vi "maincapactor11.vi"() -> ()   [LabVIEW 2020]
panel:
  out "dup directory path":path
  in  "GPIB address magnet":string="1"
  in  "GPIB address Temp Controler":string="12"
  in  "GPIB address CapBridge":string="6"
  in  "Wait (second)":u32
  in  "No of Temp Steps":i16
  in  "folder name to save files":string
  out "outputtemp":dbl[](array[numeric]) format="%.2f"
  out "outputdc":dbl[](array[numeric]) format="%.2f"
  out "outputcapacitor":dbl[](array[numeric]) format="%.2f"
  out "field":dbl[](array[numeric]) format="%.2f"
  out "Current Temp":dbl format="%.3f"
  in  "Increasing \nTemp step":bool=TRUE
  in  "Temperature\nInterval":dbl format="%.3f"
  in  "Initial Temp C":dbl format="%.3f"
  # "Help:\n1. write the folder name to save the files.The file name will \nbe the temperature in the given folder.\n2.Write the GPIB address of all the instruments before running\nthe program.\n3. Give the initial temperature and the temperature interval \nand the total number of steps.\n4.Check whether you want to increase the temperature or\ndecrease.\n5.Write the time to be waited to let the tempetature controller\nequilibrate.\n6.Once the speps 1 through 5 is done run the experiment."
  # "Decreasing\nTemp Step"
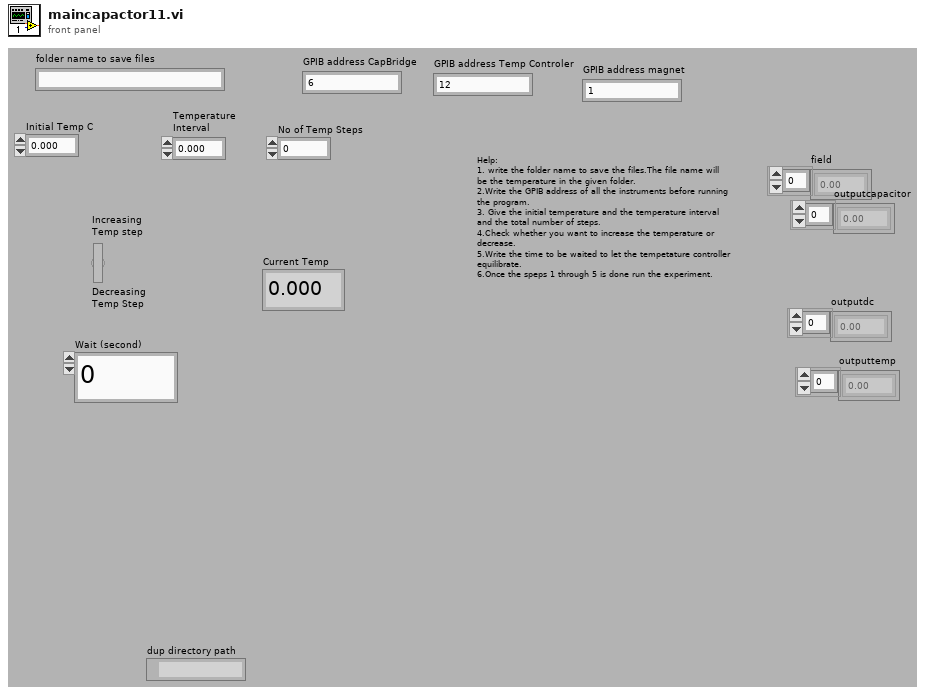
[diagram p1: front panel]
types:
  T1 = enum16{"--Quit--", "Read-Status", "Read-Cell", "Read-Field[T]", "Read-Setpoint[T]"}
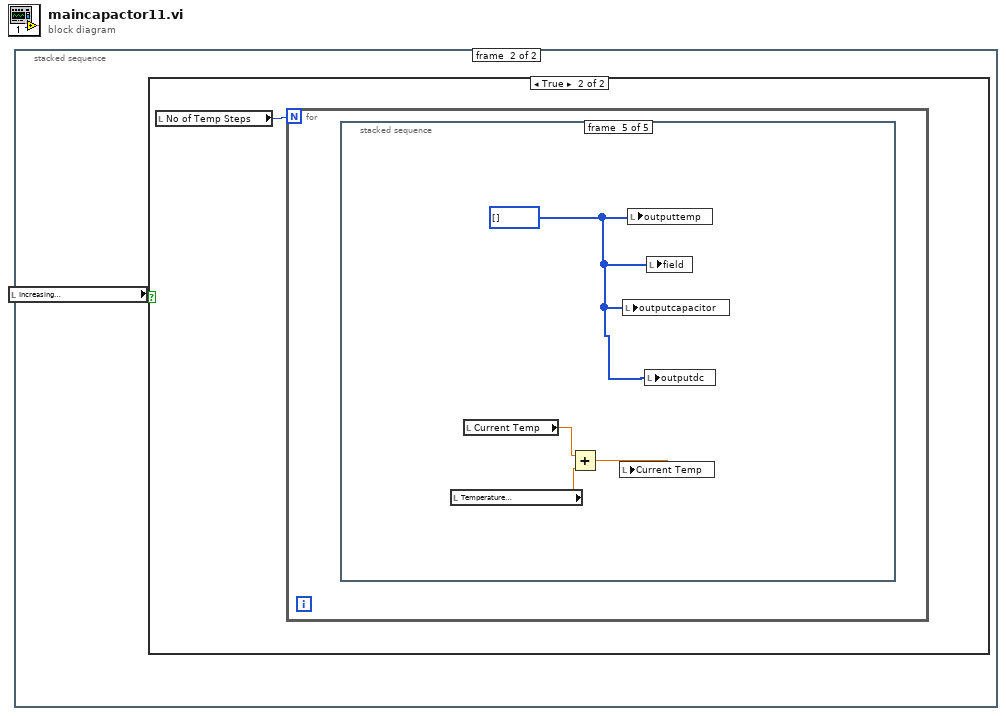
[diagram p0: block diagram]
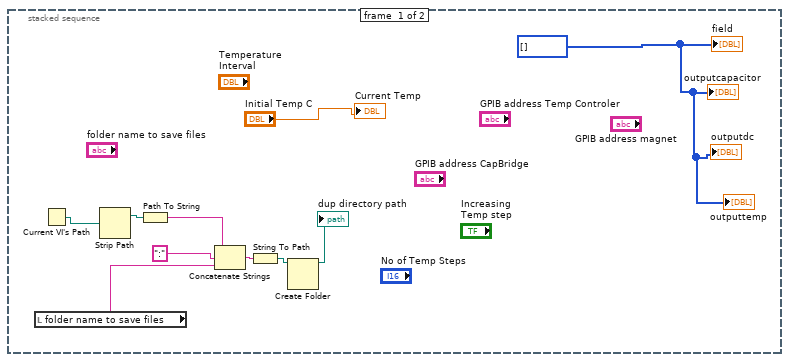
[diagram p2: hidden frame]
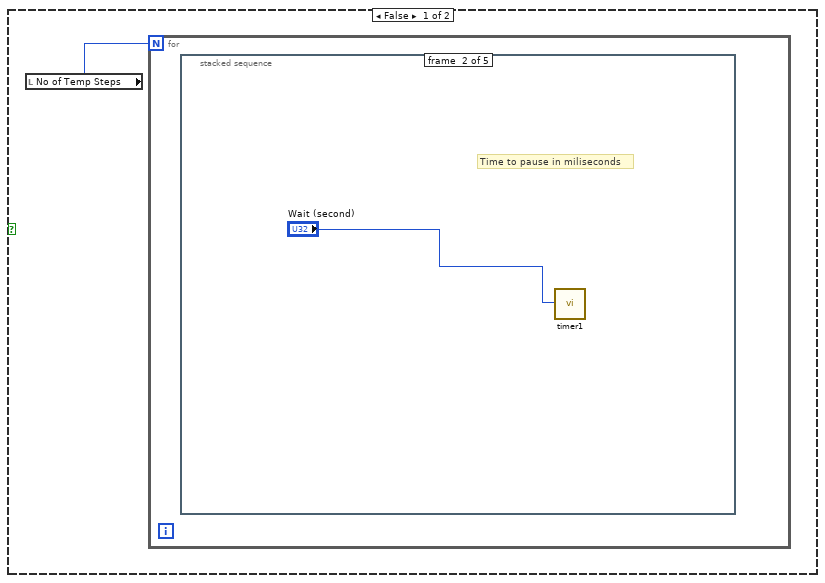
[diagram p3: hidden frame]
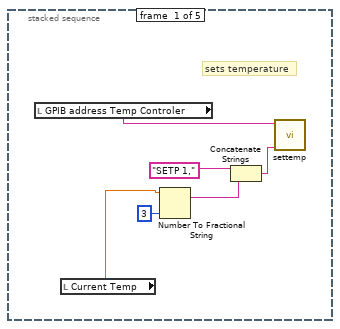
[diagram p4: hidden frame]
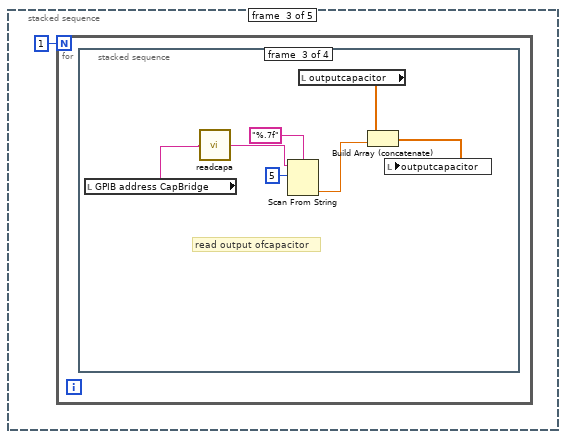
[diagram p5: hidden frame]
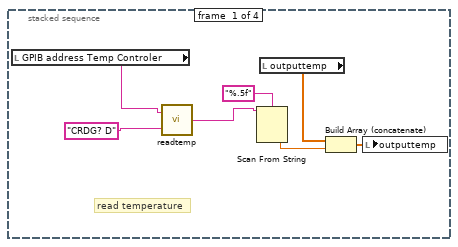
[diagram p6: hidden frame]
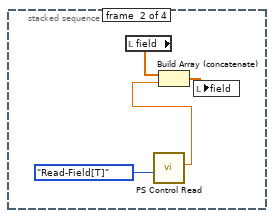
[diagram p7: hidden frame]
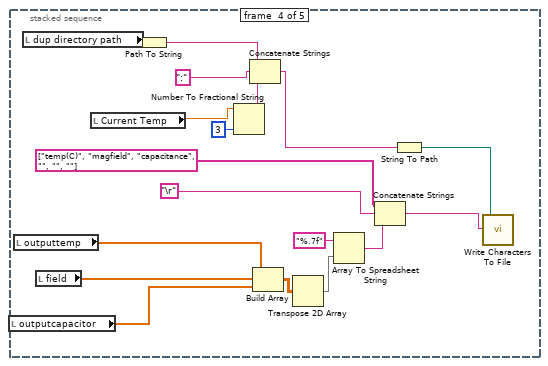
[diagram p9: hidden frame]
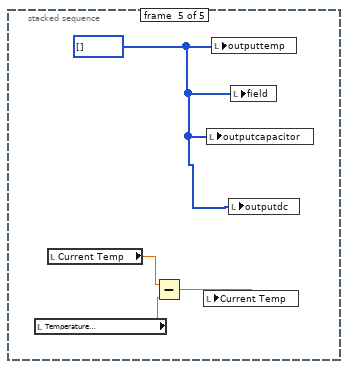
[diagram p10: hidden frame]
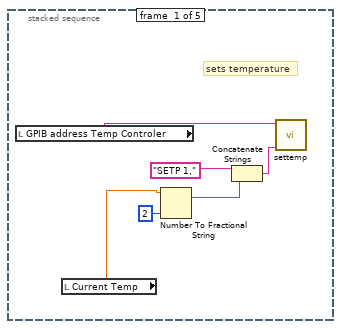
[diagram p11: hidden frame]
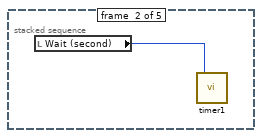
[diagram p12: hidden frame]
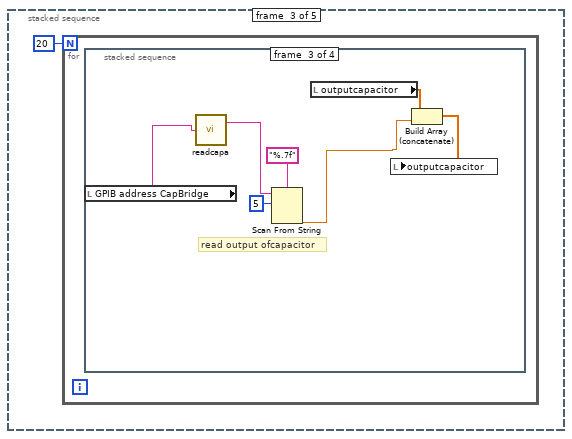
[diagram p13: hidden frame]
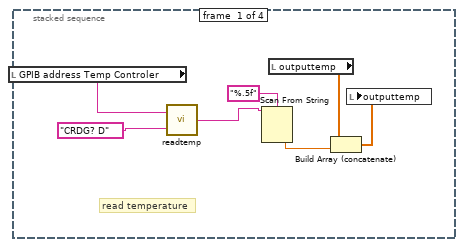
[diagram p14: hidden frame]
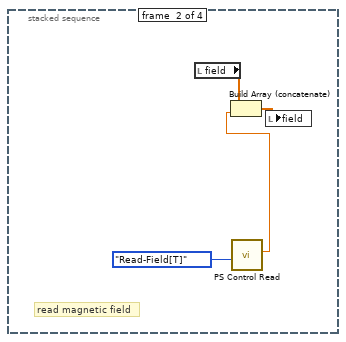
[diagram p15: hidden frame]
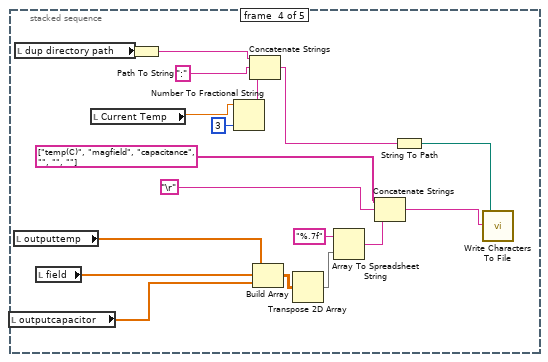
[diagram p17: hidden frame]
diagram:
  n1 = stacked-sequence {
    frame #0 {
      w9 = i32[] [] ("field")
      n2 = local read "folder name to save files"() -> (w4:string)
      n3 = Current VI's Path() -> (path=w8:path)
      n4 = Strip Path(path=w8) -> (stripped path=w7:path)  [unwired: 1 out]
      n5 = Path To String(path=w7) -> (string=w6:string)
      n6 = Concatenate Strings(w6, ":", w4) -> (w3:string)
      n7 = String To Path(string=w3) -> (path=w2:path)
      n8 = Create Folder(path (use dialog)=w2) -> (created path=→"dup directory path":path)  [unwired: 2 in, 2 out]
      "Current Temp" <- "Initial Temp C"
      "field" <- w9
      "outputcapacitor" <- w9
      "outputdc" <- w9
      "outputtemp" <- w9
    }
    frame #1 {
      n9 = local read "Increasing \nTemp step"() -> (w11:bool)
      n10 = case shown="True" w11 {
        frame False {
          n11 = local read "No of Temp Steps"() -> (w12:i16)
          n12 = for {
            N: w12 -> [_]
            n13 = stacked-sequence {
              frame #0 {
                # "sets temperature"
                n14 = local read "GPIB address Temp Controler"() -> (w13:string)
                n15 = local read "Current Temp"() -> (w15:dbl)
                n16 = Number To Fractional String(number=w15, precision (6)=i16 3) -> (F-format string=w18:string)  [unwired: 2 in]
                n17 = Concatenate Strings("SETP 1,", w18) -> (w16:string)
                n18 = call "settemp.vi"("Characters to Write"=w16, "GPIB\nAddress"=w13) -> ()  [unwired: 5 in, 1 out]
              }
              frame #1 {
                # "Time to pause in miliseconds"
                n19 = call "timer1.vi"("Numeric 2"="Wait (second)") -> ()  [unwired: 1 in]
              }
              frame #2 {
                n20 = for {
                  N: 1 -> [_]
                  n21 = stacked-sequence {
                    frame #0 {
                      # "read temperature"
                      n22 = local read "GPIB address Temp Controler"() -> (w23:string)
                      n23 = call "readtemp.vi"("Characters to Write"="CRDG? D", "GPIB\nAddress"=w23) -> ("Characters Read"=w24:string)
                      n24 = Scan From String(format string="%.5f", input string=w24) -> (output 1=w21:dbl)  [unwired: 3 in, 3 out]
                      n25 = local read "outputtemp"() -> (w22:dbl[])
                      n26 = Build Array (concatenate)(w22, w21) -> (w27:dbl[])
                      n27 = local write "outputtemp"(w27) -> ()
                    }
                    frame #1 {
                      n28 = local read "field"() -> (w30:dbl[])
                      n29 = call "PS Control Read.vi"("Read State"=T1."Read-Field[T]") -> ("Current Field"=w28:dbl)  [unwired: 3 in, 4 out]
                      n30 = Build Array (concatenate)(w30, w28) -> (w31:dbl[])
                      n31 = local write "field"(w31) -> ()
                    }
                    frame #2 {
                      # "read output ofcapacitor"
                      n32 = local read "GPIB address CapBridge"() -> (w37:string)
                      n33 = call "readcapa.vi"("GPIB\nAddress"=w37) -> ("Characters Read"=w33:string)
                      n34 = Scan From String(format string="%.7f", input string=w33, initial scan location=u32 5) -> (output 1=w32:dbl)  [unwired: 2 in, 3 out]
                      n35 = local read "outputcapacitor"() -> (w36:dbl[])
                      n36 = Build Array (concatenate)(w36, w32) -> (w38:dbl[])
                      n37 = local write "outputcapacitor"(w38) -> ()
                    }
                    frame #3 {
                      # "pause if needed"
                    }
                  }
                }
              }
              frame #3 {
                n38 = local read "outputcapacitor"() -> (w41:dbl[])
                n39 = local read "outputtemp"() -> (w51:dbl[])
                n40 = local read "dup directory path"() -> (w40:path)
                n41 = local read "field"() -> (w50:dbl[])
                n42 = local read "Current Temp"() -> (w53:dbl)
                n43 = Path To String(path=w40) -> (string=w39:string)
                n44 = Number To Fractional String(number=w53, precision (6)=i16 3) -> (F-format string=w52:string)  [unwired: 2 in]
                n45 = Concatenate Strings(w39, ":", w52) -> (w55:string)
                n46 = Build Array(w51, w50, w41) -> (w49:dbl[][])
                n47 = Transpose 2D Array(2D array=w49) -> (transposed array=w47:dbl[][])
                n48 = Array To Spreadsheet String(array=w47, 3:"%.7f" ("format string")) -> (spreadsheet string=w44:string)  [unwired: 1 in]
                n49 = Concatenate Strings(string[] ["temp(C)", "magfield", "capacitance", "", "", ""], "\r", w44) -> (w43:string)
                n50 = String To Path(string=w55) -> (path=w54:path)
                n51 = call <vilib>:"Write Characters To File.vi"("character string"=w43, "file path (dialog if empty)"=w54) -> ()  [unwired: 3 in, 1 out]
              }
              frame #4 {
                w60 = i32[] []
                n52 = local read "Temperature\nInterval"() -> (w58:dbl)
                n53 = local read "Current Temp"() -> (w59:dbl)
                n54 = Subtract(x=w59, y=w58) -> (x-y=w57:dbl)
                n55 = local write "Current Temp"(w57) -> ()
                n56 = local write "outputcapacitor"(w60) -> ()
                n57 = local write "outputtemp"(w60) -> ()
                n58 = local write "outputdc"(w60) -> ()
                n59 = local write "field"(w60) -> ()
              }
            }
          }
        }
        frame True {
          n60 = local read "No of Temp Steps"() -> (w61:i16)
          n61 = for {
            N: w61 -> [_]
            n62 = stacked-sequence {
              frame #0 {
                # "sets temperature"
                n63 = local read "GPIB address Temp Controler"() -> (w62:string)
                n64 = local read "Current Temp"() -> (w64:dbl)
                n65 = Number To Fractional String(number=w64, precision (6)=i16 2) -> (F-format string=w67:string)  [unwired: 2 in]
                n66 = Concatenate Strings("SETP 1,", w67) -> (w65:string)
                n67 = call "settemp.vi"("Characters to Write"=w65, "GPIB\nAddress"=w62) -> ()  [unwired: 5 in, 1 out]
              }
              frame #1 {
                n68 = local read "Wait (second)"() -> (w68:u32)
                n69 = call "timer1.vi"("Numeric 2"=w68) -> ()  [unwired: 1 in]
              }
              frame #2 {
                n70 = for {
                  N: 20 -> [_]
                  n71 = stacked-sequence {
                    frame #0 {
                      # "read temperature"
                      n72 = local read "GPIB address Temp Controler"() -> (w72:string)
                      n73 = call "readtemp.vi"("Characters to Write"="CRDG? D", "GPIB\nAddress"=w72) -> ("Characters Read"=w73:string)
                      n74 = Scan From String(format string="%.5f", input string=w73) -> (output 1=w70:dbl)  [unwired: 3 in, 3 out]
                      n75 = local read "outputtemp"() -> (w71:dbl[])
                      n76 = Build Array (concatenate)(w71, w70) -> (w76:dbl[])
                      n77 = local write "outputtemp"(w76) -> ()
                    }
                    frame #1 {
                      # "read magnetic field"
                      n78 = local read "field"() -> (w79:dbl[])
                      n79 = call "PS Control Read.vi"("Read State"=T1."Read-Field[T]") -> ("Current Field"=w77:dbl)  [unwired: 3 in, 4 out]
                      n80 = Build Array (concatenate)(w79, w77) -> (w80:dbl[])
                      n81 = local write "field"(w80) -> ()
                    }
                    frame #2 {
                      # "read output ofcapacitor"
                      n82 = local read "GPIB address CapBridge"() -> (w86:string)
                      n83 = call "readcapa.vi"("GPIB\nAddress"=w86) -> ("Characters Read"=w82:string)
                      n84 = Scan From String(format string="%.7f", input string=w82, initial scan location=u32 5) -> (output 1=w81:dbl)  [unwired: 2 in, 3 out]
                      n85 = local read "outputcapacitor"() -> (w85:dbl[])
                      n86 = Build Array (concatenate)(w85, w81) -> (w87:dbl[])
                      n87 = local write "outputcapacitor"(w87) -> ()
                    }
                    frame #3 {
                      # "pause if needed to take readings"
                    }
                  }
                }
              }
              frame #3 {
                n88 = local read "outputcapacitor"() -> (w90:dbl[])
                n89 = local read "outputtemp"() -> (w100:dbl[])
                n90 = local read "dup directory path"() -> (w89:path)
                n91 = local read "field"() -> (w99:dbl[])
                n92 = local read "Current Temp"() -> (w102:dbl)
                n93 = Path To String(path=w89) -> (string=w88:string)
                n94 = Number To Fractional String(number=w102, precision (6)=i16 3) -> (F-format string=w101:string)  [unwired: 2 in]
                n95 = Concatenate Strings(w88, ":", w101) -> (w104:string)
                n96 = Build Array(w100, w99, w90) -> (w98:dbl[][])
                n97 = Transpose 2D Array(2D array=w98) -> (transposed array=w96:dbl[][])
                n98 = Array To Spreadsheet String(array=w96, 3:"%.7f" ("format string")) -> (spreadsheet string=w93:string)  [unwired: 1 in]
                n99 = Concatenate Strings(string[] ["temp(C)", "magfield", "capacitance", "", "", ""], "\r", w93) -> (w92:string)
                n100 = String To Path(string=w104) -> (path=w103:path)
                n101 = call <vilib>:"Write Characters To File.vi"("character string"=w92, "file path (dialog if empty)"=w103) -> ()  [unwired: 3 in, 1 out]
              }
              frame #4 {
                w109 = i32[] []
                n102 = local read "Temperature\nInterval"() -> (w107:dbl)
                n103 = local read "Current Temp"() -> (w108:dbl)
                n104 = Add(x=w108, y=w107) -> (x+y=w106:dbl)
                n105 = local write "Current Temp"(w106) -> ()
                n106 = local write "outputcapacitor"(w109) -> ()
                n107 = local write "outputtemp"(w109) -> ()
                n108 = local write "outputdc"(w109) -> ()
                n109 = local write "field"(w109) -> ()
              }
            }
          }
        }
      }
    }
  }
